vi "Compressor TestCode.vi"(10 "Step Text":string="String") -> (2 "Compressor Output":string)   [LabVIEW 2014]
uses:
  <vilib>/Rock Robotics/WPI/Compressor/WPI_CompressorGetSetRefNum.vi
panel:
  out "Compressor Running":bool
  out "Enabled":bool
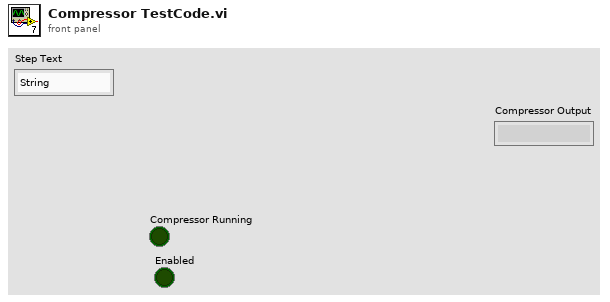
[diagram p1: front panel]
types:
  T1 = typedef "WPI_CompressorDevRef.ctl" = cluster{"DevStatus":errorcluster, "Pneumatics Control Module":u8}
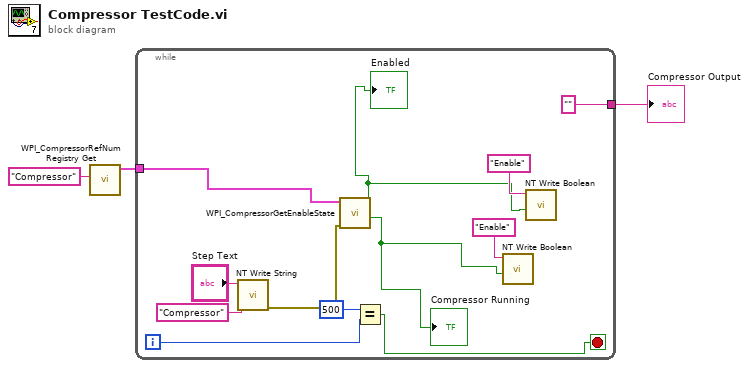
[diagram p0: block diagram]
diagram:
  n1 = call <vilib>:"WPI_CompressorRefNum Registry Get.vi"("refnum name"="Compressor") -> ("CompressorDevRef"=w2:T1)  [unwired: 9 in, 1 out]
  n2 = while {
    tunnel: w2 -> [w12]
    tunnel: ["" ("Compressor Output")] -> w1
    i -> [w10]
    stop <- w8 stop-if-true
    n3 = call <vilib>:"NT Write String.vi"("String"="Compressor", "Name"="Step Text") -> ("error out"=w15:errorcluster)  [unwired: 9 in]
    n4 = call <vilib>:"WPI_CompressorGetEnableState.vi"("error in (no error)"=w15, "CompressorDevRef"=w12) -> ("Compressor Running"=w4:bool, "Enabled"=w5:bool)  [unwired: 6 in, 2 out]
    "Enabled" <- w5
    "Compressor Running" <- w4
    n5 = Equal?(x=500, y=w10) -> (x = y?=w8:bool)
    n6 = call <vilib>:"NT Write Boolean.vi"("Boolean"=w4, "Name"="Enable") -> ()  [unwired: 9 in, 1 out]
    n7 = call <vilib>:"NT Write Boolean.vi"("Boolean"=w5, "Name"="Enable") -> ()  [unwired: 9 in, 1 out]
  }
  "Compressor Output" <- w1
